vi "CreateNamesNode.vi"(7 "DOM Document":refnum<k20>, 8 "Error In":errorcluster, 11 "Names":string[][](array[string])) -> (0 "Error Out":errorcluster, 3 "Names Node":refnum<k20>)   [LabVIEW 2012]
uses:
  libs/LV-Utilities/LV-Utilities.lvlib
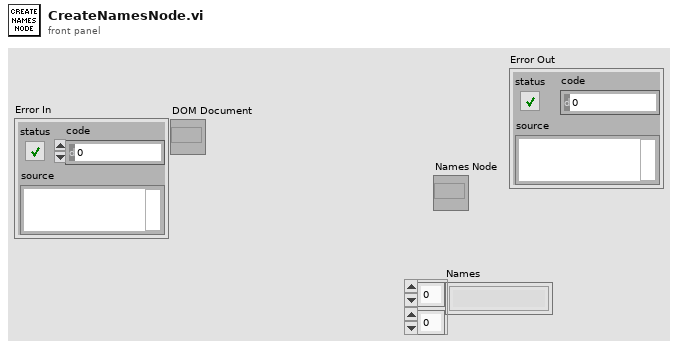
[diagram p1: front panel]
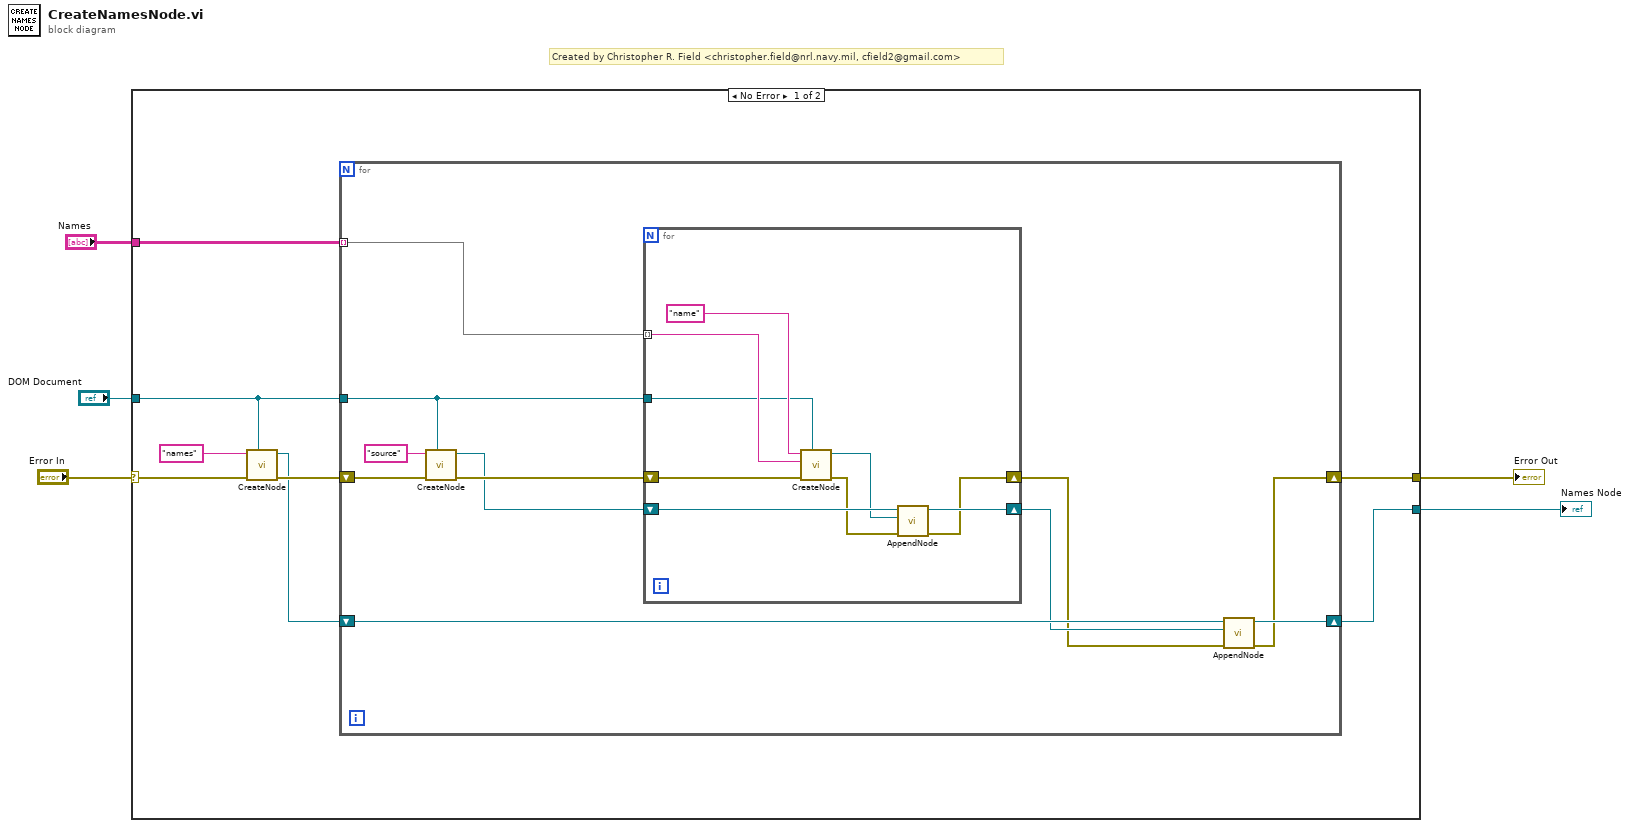
[diagram p0: block diagram]
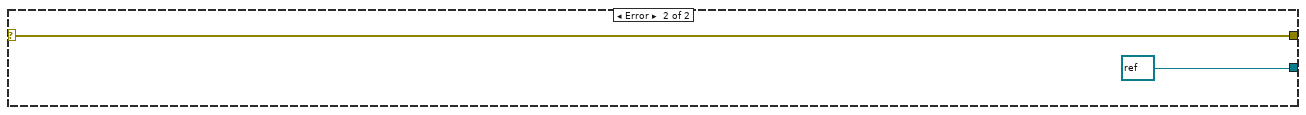
[diagram p2: hidden frame]
diagram:
  # "Created by Christopher R. Field <christopher.field@nrl.navy.mil, cfield2@gmail.com>"
  n1 = case shown="No Error" "Error In" {
    selector: "Error In" -> [w9 w35]
    tunnel: "DOM Document" -> [w6 _]
    tunnel: [w13 refnum<k20> refnum ("Wirings Node 2")] -> w3
    tunnel: [w12 w35] -> w2
    tunnel: "Names" -> [w11 _]
    frame No Error {
      n2 = call "CreateNode.vi"("DOM Document"=w6, "Error In"=w9, "Tag Name"="names") -> ("Error out"=w8:errorcluster, "Node"=w7:refnum<k20>)  [unwired: 7 in]
      n3 = for {
        shift-right: [w16] -> w12
        shift-left: w8 -> [w22]
        shift-right: [w17] -> w13
        shift-left: w7 -> [w18]
        tunnel: w11 -> [w24] mode=indexing
        tunnel: w6 -> [w19]
        n4 = call "CreateNode.vi"("DOM Document"=w19, "Error In"=w22, "Tag Name"="source") -> ("Error out"=w21:errorcluster, "Node"=w20:refnum<k20>)  [unwired: 7 in]
        n5 = for {
          shift-right: [w26] -> w14
          shift-left: w21 -> [w33]
          tunnel: w24 -> [w31] mode=indexing
          shift-right: [w27] -> w15
          shift-left: w20 -> [w30]
          tunnel: w19 -> [w25]
          n6 = call "CreateNode.vi"("DOM Document"=w25, "Error In"=w33, "Text"=w31, "Tag Name"="name") -> ("Error out"=w28:errorcluster, "Node"=w29:refnum<k20>)  [unwired: 6 in]
          n7 = call "AppendNode.vi"("Error In"=w28, "Child Node"=w29, "Parent Node In"=w30) -> ("Error Out"=w26:errorcluster, "Parent Node Out"=w27:refnum<k20>)  [unwired: 7 in]
        }
        n8 = call "AppendNode.vi"("Error In"=w14, "Child Node"=w15, "Parent Node In"=w18) -> ("Error Out"=w16:errorcluster, "Parent Node Out"=w17:refnum<k20>)  [unwired: 7 in]
      }
    }
    frame Error {
    }
  }
  "Names Node" <- w3
  "Error Out" <- w2
